vi "trigger.vi"(8 "error in (no error)":errorcluster, 11 "ILCCommunications in":refnum<class "ILCCommunications.lvclass">) -> (0 "error out":errorcluster, 3 "ILCCommunications out":refnum<class "ILCCommunications.lvclass">)   [LabVIEW 2016, in "ILCCommunications.lvclass"]
uses:
  ILCCommunications.lvclass
  ILCCommunications.lvclass/ILCCommunications.ctl
  Common_RT_FPGA/IBooleanControl/IBooleanControl.lvclass
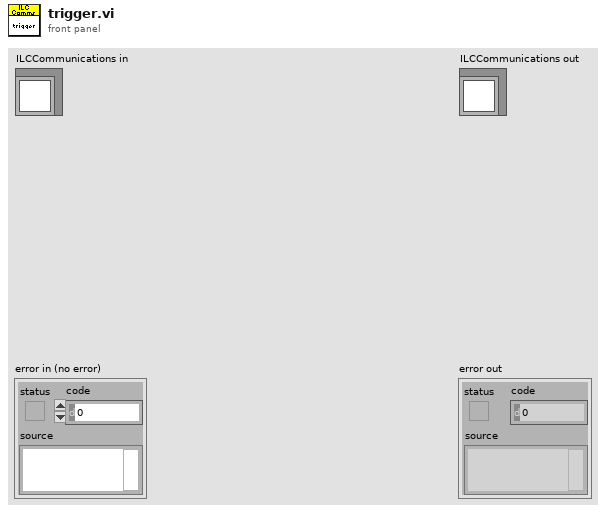
[diagram p1: front panel]
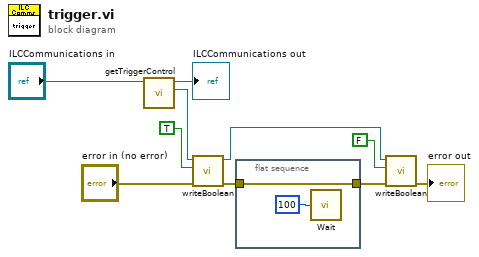
[diagram p0: block diagram]
diagram:
  n1 = call "getTriggerControl.vi"("ILCCommunications in"="ILCCommunications in") -> ("TriggerControl"=w9:refnum<class "IBooleanControl.lvclass">, "ILCCommunications out"=→"ILCCommunications out":refnum<class "ILCCommunications.lvclass">)  [unwired: 9 in]
  n2 = call-dynamic "writeBoolean.vi"("error in (no error)"="error in (no error)", "Data"=TRUE, "IBooleanControl in"=w9) -> ("error out"=w7:errorcluster, "IBooleanControl out"=w6:refnum<class "IBooleanControl.lvclass">)  [unwired: 7 in]
  n3 = flat-sequence {
    tunnel: [w12] -> w4
    tunnel: w7 -> [w12]
    frame #0 {
      n4 = call "Wait"("Count(uSec)"=u32 100) -> ()  [unwired: 1 out]
    }
  }
  n5 = call-dynamic "writeBoolean.vi"("error in (no error)"=w4, "Data"=FALSE, "IBooleanControl in"=w6) -> ("error out"=→"error out":errorcluster)  [unwired: 7 in, 1 out]
